vi "Send Change Process Params.vi"(7 "Message Priority (Normal)":T2=enum."Normal", 8 "error in (no error)":errorcluster, 10 "New Params":T1={"Mode"=enum."ROI", "Manual LUT"={"Minimum"=0.0, "Maximum"=0.0}, "BCG Values"={"Brightness"=128.0, "Contrast"=45.0, "Gamma"=1.0}, "Log?"=FALSE, "Auto?"=FALSE, "ROI"={"Global Rectangle"=[], "Contours"=[]}, "Image X"=0, "Image Y"=0, "HROI Pos"=0}, 11 "Message Enqueuer":refnum<class "Message Enqueuer.lvclass">) -> (0 "error out":errorcluster, 3 "Message Enqueuer out":refnum<class "Message Enqueuer.lvclass">)   [LabVIEW 2023, in "CameraPreview.lvlib" / "Change Process Params Msg.lvclass"]
doc: "This VI sends the message to an actor."
uses:
  Change Process Params Msg.lvclass
  <vilib>/ActorFramework/Message Enqueuer/Message Enqueuer.lvclass
  <vilib>/ActorFramework/Message Enqueuer/Message Priority.ctl
  typedefs/ImageProcessingParametersInPreview.ctl
  C:/Program Files/National Instruments/LabVIEW 2023/vi.lib/ActorFramework/Message/Message.lvclass
  Change Process Params Msg.lvclass/Change Process Params Msg.ctl
  <vilib>/ActorFramework/Message Enqueuer/Message Enqueuer.lvclass/Message Enqueuer.ctl
  <vilib>/ActorFramework/Message Priority Queue/Priority Enqueue.vi
  C:/Users/quantum/Documents/LVDAQ/UIs/Camera_Preview/CameraPreview/CameraPreview Messages/Change Process Params Msg/Change Process Params Msg.lvclass
  typedefs/typedefs.lvlib
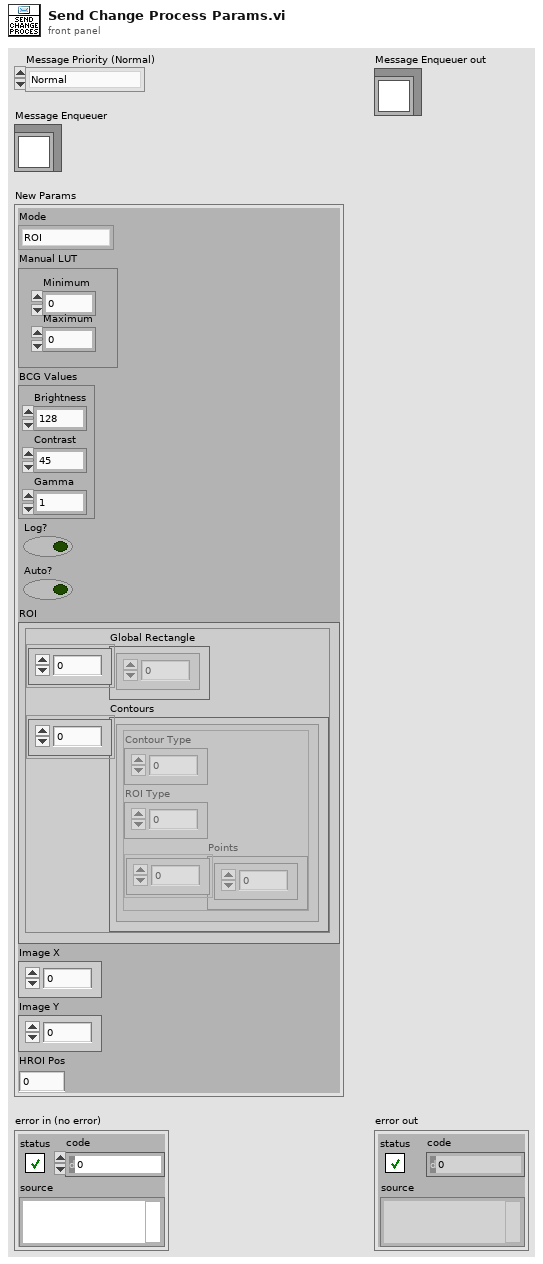
[diagram p1: front panel]
types:
  T1 = typedef "typedefs.lvlib/ImageProcessingParametersInPreview.ctl" = cluster{"Mode":enum16{"ROI", "Image"}, "Manual LUT":cluster{"Minimum":dbl, "Maximum":dbl}, "BCG Values":cluster{"Brightness":sgl, "Contrast":sgl, "Gamma":sgl}, "Log?":bool, "Auto?":bool, "ROI":cluster{"Global Rectangle":i32[], "Contours":cluster{"Contour Type":u32, "ROI Type":u32, "Points":i32[]}[]}, "Image X":i32, "Image Y":i32, "HROI Pos":u16}
  T2 = typedef "Actor Framework.lvlib/Message Enqueuer.lvclass/Message Priority.ctl" = enum16{"Low", "Normal", "High"}
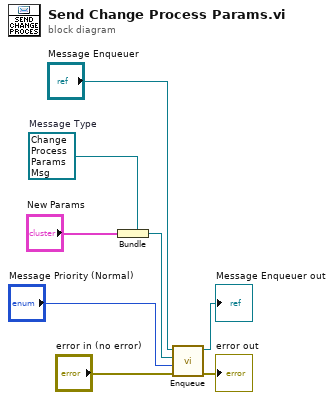
[diagram p0: block diagram]
diagram:
  w5 = refnum<class "Change Process Params Msg.lvclass"> refnum  # Message Type
  n1 = Bundle(cluster=w5, "New Params") -> (w4:refnum<class "Change Process Params Msg.lvclass">)
  n2 = call <vilib>:"Enqueue.vi"("error in (no error)"="error in (no error)", "Message Priority (Normal)"="Message Priority (Normal)", "Message"=w4, "Message Enqueuer in"="Message Enqueuer") -> ("error out"=→"error out":errorcluster, "Message Enqueuer in"=→"Message Enqueuer out":refnum<class "Message Enqueuer.lvclass">)  [unwired: 6 in]
